vi "Populate Line Numbers.vi"(0 "Line Numbers in":refnum<vi>, 7 "Total Number of Lines":i32) -> (4 "Line Numbers out":refnum<vi>)   [LabVIEW 2016, in "Code String LV.lvclass"]
doc: "Populates <b>Line Numbers</b> with numbers.\nIf the current number of lines in <b>Line Numbers</b> is less than <b>Total Number of Lines</b>, new items will be added; if greater, lines will be subtracted. If 0, <b>Line Numbers</b> is cleared.\n--------------------\nCopyright (c) 2019 Analog Devices, Inc. All rights reserved.\n\nRedistribution and use in source and binary forms, with or without modification,\nare permitted provided that the following conditions are met:\n - Redistributions of source code must retain the above copyright notice, this\n list of conditions and the following disclaimer.\n - Redistributions in binary form must reproduce the above copyright notice,\n this list of conditions and the following disclaimer in the documentation\n and/or other materials provided with the distribution.\n - Modified versions of the software must be conspicuously marked as such.\n - This software is licensed solely and exclusively for use with\n processors/products manufactured by or for Analog Devices, Inc.\n - This software may not be combined or merged with other code in any manner\n that would cause the software to become subject to terms and conditions\n which differ from those listed here.\n - Neither the name of Analog Devices, Inc. nor the names of its contributors\n may be used to endorse or promote products derived from this software\n without specific prior written permission.\n - The use of this software may or may not infringe the patent rights of one or\n more patent holders. This license does not release you from the requirement\n that you obtain separate licenses from these patent holders to use this\n software.\n\nTHIS SOFTWARE IS PROVIDED BY ANALOG DEVICES, INC. AND CONTRIBUTORS \"AS IS\" AND\nANY EXPRESS OR IMPLIED WARRANTIES, INCLUDING, BUT NOT LIMITED TO,\nNON-INFRINGEMENT, TITLE, MERCHANTABILITY AND FITNESS FOR A PARTICULAR PURPOSE\nARE DISCLAIMED. IN NO EVENT SHALL ANALOG DEVICES, INC. OR CONTRIBUTORS BE LIABLE\nFOR ANY DIRECT, INDIRECT, INCIDENTAL, SPECIAL, EXEMPLARY, PUNITIVE OR\nCONSEQUENTIAL DAMAGES (INCLUDING, BUT NOT LIMITED TO, DAMAGES ARISING OUT OF\nCLAIMS OF INTELLECTUAL PROPERTY RIGHTS INFRINGEMENT; PROCUREMENT OF SUBSTITUTE\nGOODS OR SERVICES; LOSS OF USE, DATA, OR PROFITS; OR BUSINESS INTERRUPTION)\nHOWEVER CAUSED AND ON ANY THEORY OF LIABILITY, WHETHER IN CONTRACT, STRICT\nLIABILITY, OR TORT (INCLUDING NEGLIGENCE OR OTHERWISE) ARISING IN ANY WAY OUT OF\nTHE USE OF THIS SOFTWARE, EVEN IF ADVISED OF THE POSSIBILITY OF SUCH DAMAGE.\n\n2019-01-10-7CBSD SLA"
uses:
  Code String LV.lvclass
panel:
  # "Copyright (c) 2019 Analog Devices, Inc.  All rights reserved.\n\nRedistribution and use in source and binary forms, with or without modification,\nare permitted provided that the following conditions are met:\n  - Redistributions of source code must retain the above copyright notice, this\n    list of conditions and the following disclaimer.\n  - Redistributions in binary form must reproduce the above copyright notice,\n    this list of conditions and the following disclaimer in the documentation\n    and/or other materials provided with the distribution.\n  - Modified versions of the software must be conspicuously marked as such.\n  - This software is licensed solely and exclusively for use with\n    processors/products manufactured by or for Analog Devices, Inc.\n  - This software may not be combined or merged with other code in any manner\n    that would cause the software to become subject to terms and conditions\n    which differ from those listed here.\n  - Neither the name of Analog Devices, Inc. nor the names of its contributors\n    may be used to endorse or promote products derived from this software\n    without specific prior written permission.\n  - The use of this software may or may not infringe the patent rights of one or\n    more patent holders.  This license does not release you from the requirement\n    that you obtain separate licenses from these patent holders to use this\n    software.\n\nTHIS SOFTWARE IS PROVIDED BY ANALOG DEVICES, INC. AND CONTRIBUTORS \"AS IS\" AND\nANY EXPRESS OR IMPLIED WARRANTIES, INCLUDING, BUT NOT LIMITED TO,\nNON-INFRINGEMENT, TITLE, MERCHANTABILITY AND FITNESS FOR A PARTICULAR PURPOSE\nARE DISCLAIMED. IN NO EVENT SHALL ANALOG DEVICES, INC. OR CONTRIBUTORS BE LIABLE\nFOR ANY DIRECT, INDIRECT, INCIDENTAL, SPECIAL, EXEMPLARY, PUNITIVE OR\nCONSEQUENTIAL DAMAGES (INCLUDING, BUT NOT LIMITED TO, DAMAGES ARISING OUT OF\nCLAIMS OF INTELLECTUAL PROPERTY RIGHTS INFRINGEMENT; PROCUREMENT OF SUBSTITUTE\nGOODS OR SERVICES; LOSS OF USE, DATA, OR PROFITS; OR BUSINESS INTERRUPTION)\nHOWEVER CAUSED AND ON ANY THEORY OF LIABILITY, WHETHER IN CONTRACT, STRICT\nLIABILITY, OR TORT (INCLUDING NEGLIGENCE OR OTHERWISE) ARISING IN ANY WAY OUT OF\nTHE USE OF THIS SOFTWARE, EVEN IF ADVISED OF THE POSSIBILITY OF SUCH DAMAGE.\n\n2019-01-10-7CBSD SLA"
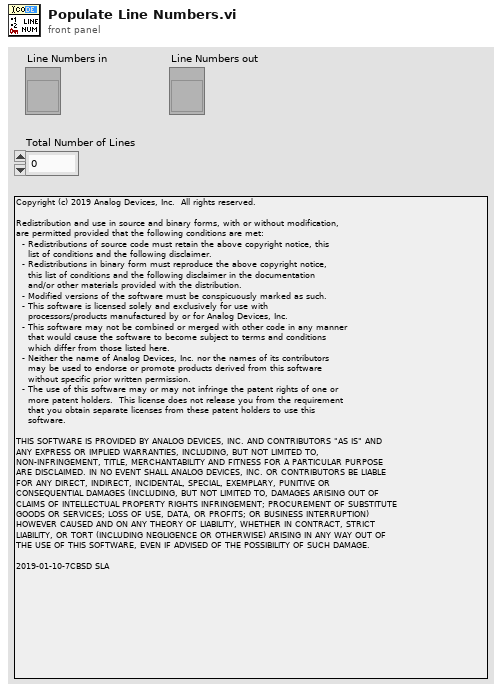
[diagram p1: front panel]
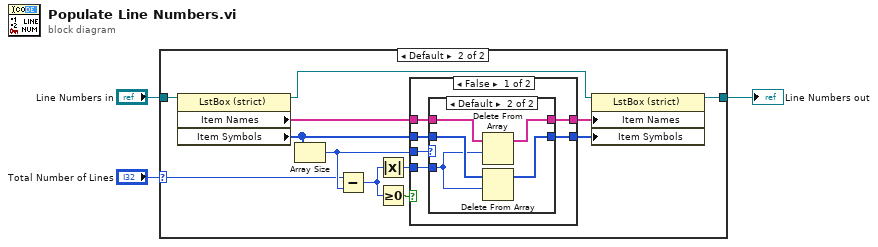
[diagram p0: block diagram]
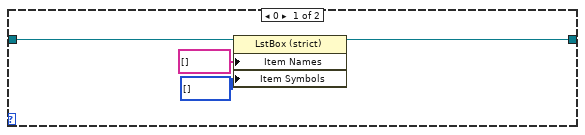
[diagram p2: hidden frame]
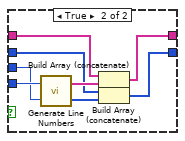
[diagram p4: hidden frame]
diagram:
  n1 = case shown="Default" "Total Number of Lines" {
    selector: "Total Number of Lines" -> [_ w13]
    tunnel: "Line Numbers in" -> [w7 w19]
    tunnel: [w6 w9] -> w2
    frame 0 {
      n2 = property class="LstBox (strict)"(reference=w7, "Item Names"=string[] [], "Item Symbols"=i32[] []) -> (reference out=w6:refnum<vi>)  [unwired: 1 in, 1 out]
    }
    frame Default {
      n3 = property class="LstBox (strict)"(reference=w19) -> (reference out=w10:refnum<vi>, "Item Names"=w18:string[], "Item Symbols"=w17:i32[])  [unwired: 1 in, 1 out]
      n4 = Array Size(array=w17) -> (size(s)=w16:i32)
      n5 = Subtract(x=w13, y=w16) -> (x-y=w14:i32)
      n6 = Absolute Value(x=w14) -> (abs(x)=w8:i32)
      n7 = Greater Or Equal To 0?(x=w14) -> (x >= 0?=w15:bool)
      n8 = case shown="False" w15 {
        tunnel: w18 -> [w25 w40]
        tunnel: [w22 w39] -> w12
        tunnel: [w21 w38] -> w11
        tunnel: w8 -> [w24 w35]
        tunnel: w17 -> [w23 w34]
        tunnel: w16 -> [w20 w33]
        frame False {
          n9 = case shown="Default" w20 {
            tunnel: w25 -> [w26 w32]
            tunnel: w24 -> [_ w28]
            tunnel: w23 -> [w27 w31]
            tunnel: [w26 w30] -> w22
            tunnel: [w27 w29] -> w21
            frame 1 {
            }
            frame Default {
              n10 = Delete From Array(array=w32, length=w28) -> (array with subset deleted=w30:string[])  [unwired: 1 in, 1 out]
              n11 = Delete From Array(array=w31, length=w28) -> (array with subset deleted=w29:i32[])  [unwired: 1 in, 1 out]
            }
          }
        }
        frame True {
          n12 = call "Generate Line Numbers.vi"("Offset (0)"=w33, "Number of Items"=w35) -> ("Symbols"=w36:i32[], "Numeric List"=w37:string[])
          n13 = Build Array (concatenate)(w40, w37) -> (w39:string[])
          n14 = Build Array (concatenate)(w34, w36) -> (w38:i32[])
        }
      }
      n15 = property class="LstBox (strict)"(reference=w10, "Item Names"=w12, "Item Symbols"=w11) -> (reference out=w9:refnum<vi>)  [unwired: 1 in, 1 out]
    }
  }
  "Line Numbers out" <- w2
